vi "Wolna_wydziel analogowe.vi"(8 "error in (no error)":errorcluster, 10 "Kanaly in":i32[](array[numeric]), 11 "Analogowe in":waveform(dbl)[](array[waveform])) -> (0 "error out":errorcluster, 2 "wybrany 2":waveform(dbl), 3 "wybrany 1":waveform(dbl))   [LabVIEW 2013]
doc: "Wydziala wybrane numery kanalow.\nSprawdza długość wektora kanałów,\njeżeli jest 1 to wydziela dwa te same kanaly\njeżeli jest 2 to wydziela dwa różne kanaly"
panel:
  out "Kanaly out":i32[](array[numeric])
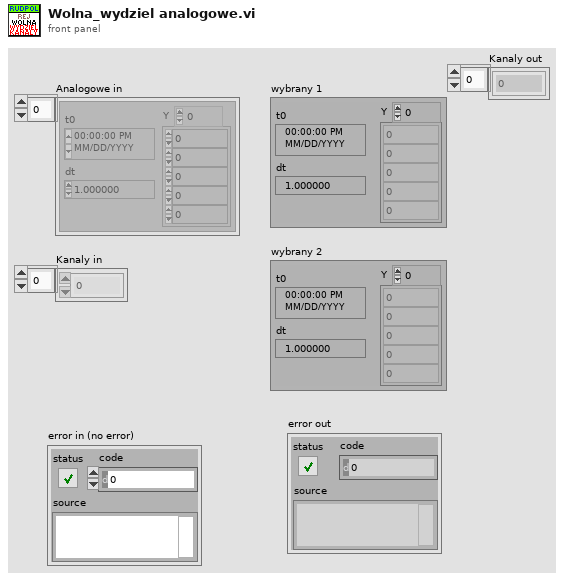
[diagram p1: front panel]
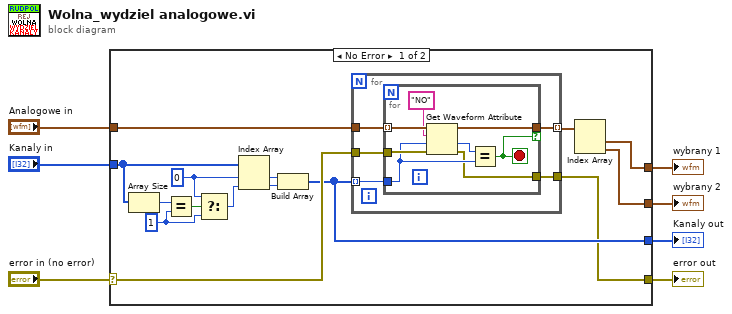
[diagram p0: block diagram]
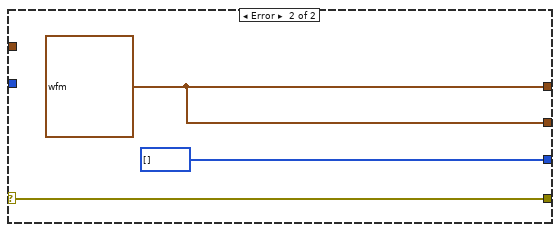
[diagram p2: hidden frame]
diagram:
  n1 = case shown="No Error" "error in (no error)" {
    selector: "error in (no error)" -> [w13 w37]
    tunnel: "Kanaly in" -> [w22 _]
    tunnel: [w9 w38] -> w6
    tunnel: [w10 w38] -> w5
    tunnel: "Analogowe in" -> [w15 _]
    tunnel: [w8 w37] -> w2
    tunnel: [w12 i32[] []] -> w1
    frame No Error {
      w19 = 0 ("y")
      w17 = 1 ("y")
      n2 = Array Size(array=w22) -> (size(s)=w21:i32)
      n3 = Equal?(x=w21, y=w17) -> (x = y?=w20:bool)
      n4 = Select(t=w19, s=w20, f=w17) -> (s? t:f=w18:i32)
      n5 = Index Array(array=w22, index #1=w19, index #2=w18) -> (element #1=w14:i32, element #2=w16:i32)
      n6 = Build Array(w14, w16) -> (w12:i32[])
      n7 = for {
        tunnel: w15 -> [w27]
        tunnel: w12 -> [w26] mode=indexing
        tunnel: w13 -> [w25]
        tunnel: [w24] -> w11 mode=indexing
        tunnel: [w23] -> w8
        n8 = for {
          tunnel: w27 -> [w35] mode=indexing
          tunnel: w26 -> [w30]
          tunnel: [w34] -> w24 if=w29
          tunnel: w25 -> [w32]
          tunnel: [w28] -> w23
          stop <- w29 stop-if-true
          n9 = Get Waveform Attribute(4:w32, 5:w30, 6:"NO" ("name"), 7:w35) -> (0:w28:errorcluster, 1:w31:i32, 3:w34:waveform(dbl))  [unwired: 1 out]
          n10 = Equal?(x=w31, y=w30) -> (x = y?=w29:bool)
        }
      }
      n11 = Index Array(array=w11) -> (element #1=w10:waveform(dbl), element #2=w9:waveform(dbl))  [unwired: 2 in]
    }
    frame Error {
      w38 = waveform(dbl) {"t0"=timestamp(0 s since 1904-01-01), "dt"=1.0, "Y"=[]} ("Waveform")
    }
  }
  "wybrany 2" <- w6
  "wybrany 1" <- w5
  "error out" <- w2
  "Kanaly out" <- w1
